vi "Motic Get Binning List.vi"(8 "error in (no error)":errorcluster, 10 "binning count":i32, 11 "camera":i32) -> (0 "error out":errorcluster, 1 "height array out":i32[](array[numeric]), 2 "width array out":i32[](array[numeric]), 3 "camera out":i32)   [LabVIEW 2012, in "MoticApi.lvlib"]
doc: "MOTICAPI bool Motic_getBinningList(MUCam_Handle camera, int *w, int *h);"
uses:
  MoticApi.lvlib
  MoticApi.dll
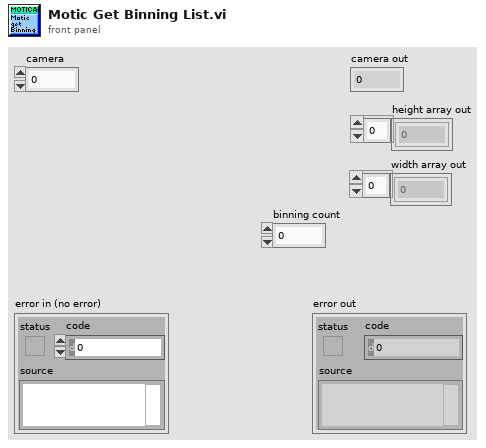
[diagram p1: front panel]
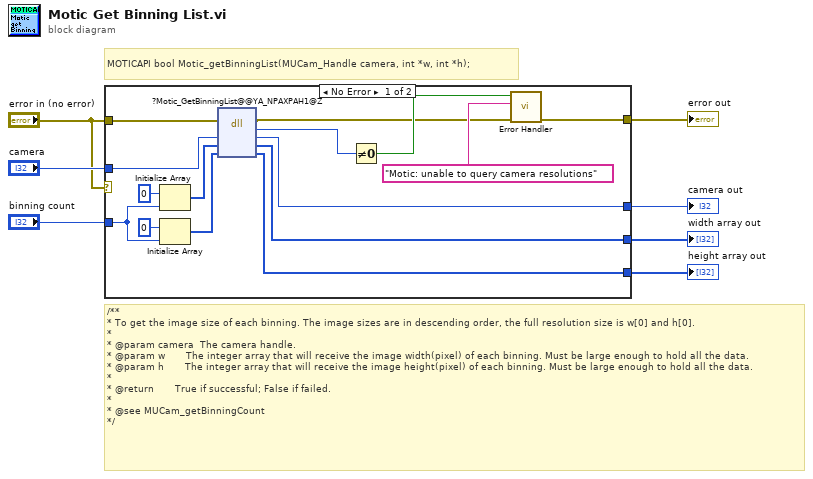
[diagram p0: block diagram]
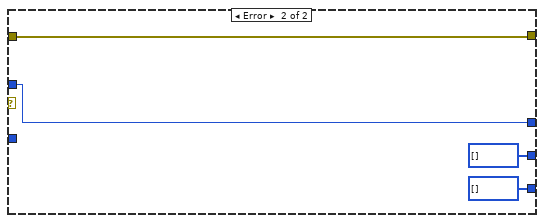
[diagram p2: hidden frame]
diagram:
  # "/**\n* To get the image size of each binning. The image sizes are in descending order, the full resolution size is w[0] and h[0].\n*\n* @param camera  The camera handle.\n* @param w       The integer array that will receive the image width(pixel) of each binning. Must be large enough to hold all the data.\n* @param h       The integer array that will receive the image height(pixel) of each binning. Must be large enough to hold all the data.\n*\n* @return       True if successful; False if failed.\n*\n* @see MUCam_getBinningCount\n*/"
  # "MOTICAPI bool Motic_getBinningList(MUCam_Handle camera, int *w, int *h);"
  n1 = case shown="No Error" "error in (no error)" {
    tunnel: "camera" -> [w21 w25]
    tunnel: [w20 w25] -> w6
    tunnel: "error in (no error)" -> [w19 w26]
    tunnel: [w18 i32[] [] ("width array")] -> w5
    tunnel: [w17 i32[] [] ("height array")] -> w4
    tunnel: "binning count" -> [w14 _]
    tunnel: [w11 w26] -> w2
    frame No Error {
      n2 = Initialize Array(0 ("element"), w14) -> (w13:i32[])
      n3 = Initialize Array(0 ("element"), w14) -> (w12:i32[])
      n4 = dll-call lib="C:/Users/TTS-Digital/Desktop/MoticApi/MoticApi_git/MoticApi/MoticApi.*" fn="?Motic_GetBinningList@@YA_NPAXPAH1@Z"(error in=w19, "camera"=w21, "width array"=w13, "height array"=w12) -> (error out=w8:errorcluster, "return type"=w22:u8, "camera"=w20:i32, "width array"=w18:i32[], "height array"=w17:i32[])  [unwired: 2 in, 1 out]
      n5 = Not Equal To 0?(x=w22) -> (x != 0?=w10:bool)
      n6 = call "Error Handler.vi"("error in (no error)"=w8, "Error message"="Motic: unable to query camera resolutions" ("source"), "Function return"=w10) -> ("error out"=w11:errorcluster)  [unwired: 8 in]
    }
    frame Error {
    }
  }
  "camera out" <- w6
  "error out" <- w2
  "width array out" <- w5
  "height array out" <- w4
